vi "Compare Parameters.vi"(9 "refresh listbox":T4[](array[typedef]), 10 "new parameter":T1={"name"="", "unit"="", "Parameter"={"start index"=0, "size"=1, "encoding"=enum."BNR", "signed"=FALSE, "scale multiplier"=1.0, "scale offset"=0.0, "default value"=0.0}}, 11 "old parameter":T1={"name"="", "unit"="", "Parameter"={"start index"=0, "size"=1, "encoding"=enum."BNR", "signed"=FALSE, "scale multiplier"=1.0, "scale offset"=0.0, "default value"=0.0}}) -> (1 "refresh listbox out":T4[](array[typedef]), 2 "any changes?":bool)   [LabVIEW 2024, in "AIM ARINC 429 System Explorer.lvlib" / "Implementation.lvlib"]
uses:
  Implementation.lvlib
  Types/Refresh Listbox.ctl
  Types/Refresh Symbols.ctl
  Shared/VS Channel Definition for Parameter.ctl
  Shared/Parameter Definition.ctl
  <vilib>/NI/NI VeriStand Encoding and Decoding/Encoding.ctl
  Refresh Constants.vi
  <vilib>/NI/NI VeriStand Encoding and Decoding/Encoding and Decoding.lvlib
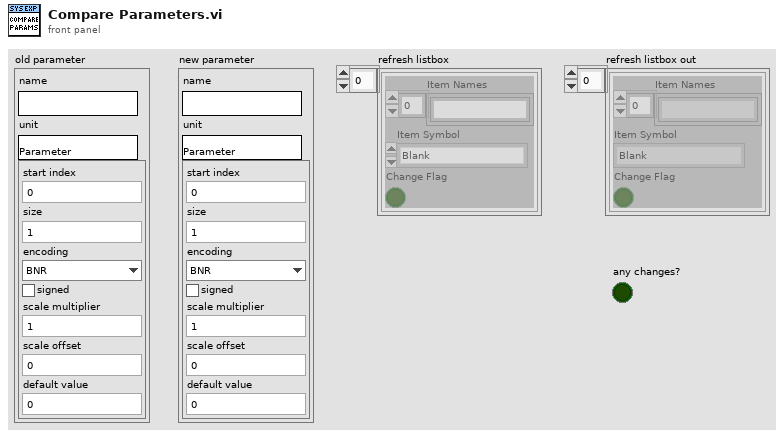
[diagram p1: front panel]
types:
  T1 = typedef "VS Channel Definition for Parameter.ctl" = cluster{"name":string, "unit":string, "Parameter":T2}
  T2 = typedef "Parameter Definition.ctl" = cluster{"start index":i32, "size":i32, "encoding":T3, "signed":bool, "scale multiplier":dbl, "scale offset":dbl, "default value":dbl}
  T3 = typedef "Encoding and Decoding.lvlib/Encoding.ctl" = enum16{"BNR", "BCD", "Discrete"}
  T4 = typedef "AIM ARINC 429 System Explorer.lvlib/Implementation.lvlib/Refresh Listbox.ctl" = cluster{"Item Names":string[], "Item Symbol":T5, "Change Flag":bool}
  T5 = typedef "AIM ARINC 429 System Explorer.lvlib/Implementation.lvlib/Refresh Symbols.ctl" = enum16{"Blank", "Port", "Incoming", "Outgoing", "Label", "Word", "Parameter", "ARINC-429", "Config Files", "Channel Spec", "Item"}
  T6 = cluster{"name":bool, "unit":bool, "Parameter":cluster{"start index":bool, "size":bool, "encoding":bool, "signed":bool, "scale multiplier":bool, "scale offset":bool, "default value":bool}}
  T7 = typedef "AIM ARINC 429 System Explorer.lvlib/Implementation.lvlib/Parameter Strings.ctl" = cluster{"name":string, "default value":string, "unit":string, "start index":string, "size":string, "encoding":string, "signed":string, "scale multiplier":string, "scale offset":string}
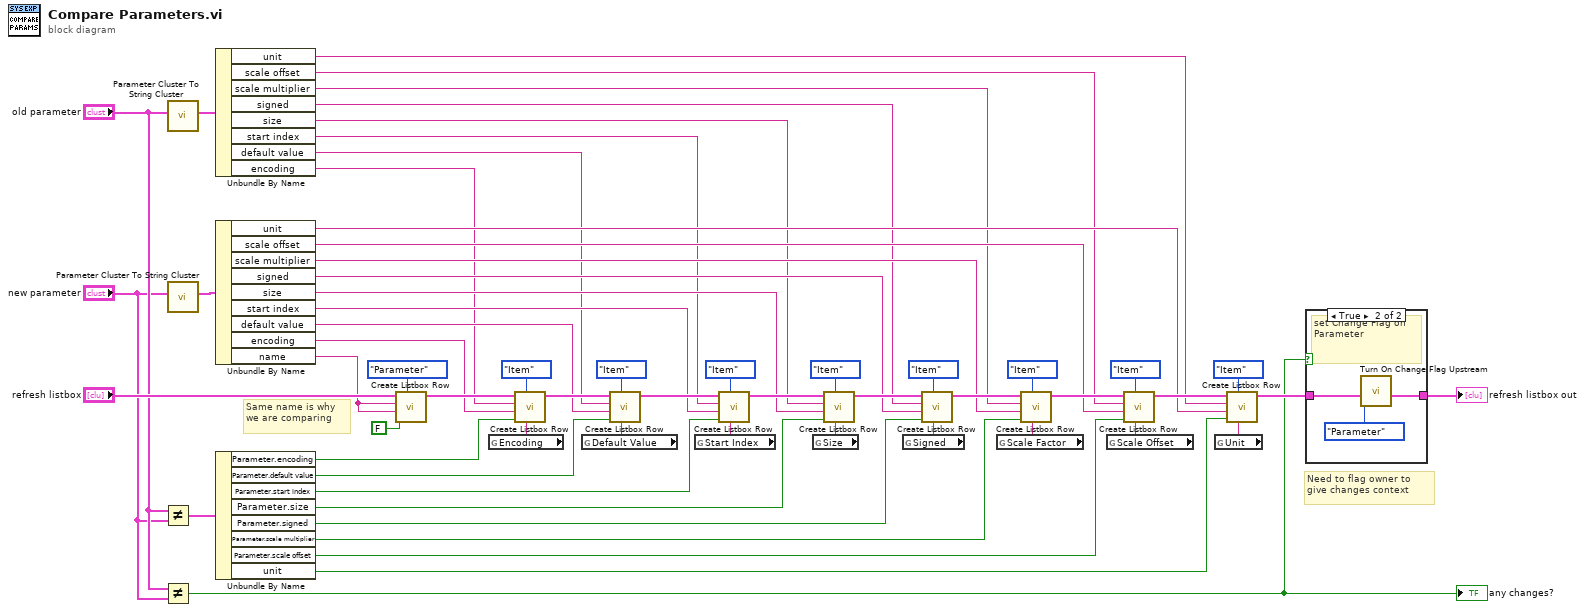
[diagram p0: block diagram]
diagram:
  # "Need to flag owner to give changes context"
  # "Same name is why we are comparing"
  n1 = Not Equal?(x="old parameter", y="new parameter") -> (x != y?=w14:T6)
  n2 = Not Equal?(x="old parameter", y="new parameter") -> (x != y?=w1:bool)
  "any changes?" <- w1
  n3 = call "Parameter Cluster To String Cluster.vi"("parameter"="old parameter") -> ("parameter strings"=w31:T7)  [unwired: 10 in]
  n4 = call "Parameter Cluster To String Cluster.vi"("parameter"="new parameter") -> ("parameter strings"=w41:T7)  [unwired: 10 in]
  n5 = Unbundle By Name(w31) -> ("unit"=w23:string, "scale offset"=w24:string, "scale multiplier"=w25:string, "signed"=w26:string, "size"=w27:string, "start index"=w28:string, "default value"=w29:string, "encoding"=w30:string)
  n6 = Unbundle By Name(w41) -> ("unit"=w32:string, "scale offset"=w33:string, "scale multiplier"=w34:string, "signed"=w35:string, "size"=w36:string, "start index"=w37:string, "default value"=w38:string, "encoding"=w39:string, "name"=w40:string)
  n7 = Unbundle By Name(w14) -> ("Parameter.encoding"=w13:bool, "Parameter.default value"=w12:bool, "Parameter.start index"=w11:bool, "Parameter.size"=w10:bool, "Parameter.signed"=w9:bool, "Parameter.scale multiplier"=w8:bool, "Parameter.scale offset"=w7:bool, "unit"=w6:bool)
  n8 = call "Create Listbox Row.vi"("refresh symbol (Blank)"=Refresh_Symbols."Parameter" ("Refresh Symbol (Blank)"), "change? (T)"=FALSE, "new item"=w40, "old item"=w40, "refresh listbox"="refresh listbox") -> ("refresh listbox out"=w57:T4[])  [unwired: 6 in]
  n9 = global read "Refresh Constants.vi" "Encoding"() -> (w22:string)
  n10 = call "Create Listbox Row.vi"("override name"=w22, "refresh symbol (Blank)"=Refresh_Symbols."Item" ("Refresh Symbol (Blank)"), "change? (T)"=w13, "new item"=w39, "old item"=w30, "refresh listbox"=w57) -> ("refresh listbox out"=w55:T4[])  [unwired: 5 in]
  n11 = global read "Refresh Constants.vi" "Default Value"() -> (w15:string)
  n12 = call "Create Listbox Row.vi"("override name"=w15, "refresh symbol (Blank)"=Refresh_Symbols."Item" ("Refresh Symbol (Blank)"), "change? (T)"=w12, "new item"=w38, "old item"=w29, "refresh listbox"=w55) -> ("refresh listbox out"=w53:T4[])  [unwired: 5 in]
  n13 = global read "Refresh Constants.vi" "Start Index"() -> (w16:string)
  n14 = call "Create Listbox Row.vi"("override name"=w16, "refresh symbol (Blank)"=Refresh_Symbols."Item" ("Refresh Symbol (Blank)"), "change? (T)"=w11, "new item"=w37, "old item"=w28, "refresh listbox"=w53) -> ("refresh listbox out"=w51:T4[])  [unwired: 5 in]
  n15 = global read "Refresh Constants.vi" "Size"() -> (w17:string)
  n16 = call "Create Listbox Row.vi"("override name"=w17, "refresh symbol (Blank)"=Refresh_Symbols."Item" ("Refresh Symbol (Blank)"), "change? (T)"=w10, "new item"=w36, "old item"=w27, "refresh listbox"=w51) -> ("refresh listbox out"=w49:T4[])  [unwired: 5 in]
  n17 = global read "Refresh Constants.vi" "Signed"() -> (w18:string)
  n18 = call "Create Listbox Row.vi"("override name"=w18, "refresh symbol (Blank)"=Refresh_Symbols."Item" ("Refresh Symbol (Blank)"), "change? (T)"=w9, "new item"=w35, "old item"=w26, "refresh listbox"=w49) -> ("refresh listbox out"=w47:T4[])  [unwired: 5 in]
  n19 = global read "Refresh Constants.vi" "Scale Factor"() -> (w19:string)
  n20 = call "Create Listbox Row.vi"("override name"=w19, "refresh symbol (Blank)"=Refresh_Symbols."Item" ("Refresh Symbol (Blank)"), "change? (T)"=w8, "new item"=w34, "old item"=w25, "refresh listbox"=w47) -> ("refresh listbox out"=w45:T4[])  [unwired: 5 in]
  n21 = global read "Refresh Constants.vi" "Scale Offset"() -> (w20:string)
  n22 = call "Create Listbox Row.vi"("override name"=w20, "refresh symbol (Blank)"=Refresh_Symbols."Item" ("Refresh Symbol (Blank)"), "change? (T)"=w7, "new item"=w33, "old item"=w24, "refresh listbox"=w45) -> ("refresh listbox out"=w43:T4[])  [unwired: 5 in]
  n23 = global read "Refresh Constants.vi" "Unit"() -> (w21:string)
  n24 = call "Create Listbox Row.vi"("override name"=w21, "refresh symbol (Blank)"=Refresh_Symbols."Item" ("Refresh Symbol (Blank)"), "change? (T)"=w6, "new item"=w32, "old item"=w23, "refresh listbox"=w43) -> ("refresh listbox out"=w5:T4[])  [unwired: 5 in]
  n25 = case shown="True" w1 {
    tunnel: w5 -> [w61 w64]
    tunnel: [w61 w62] -> w4
    frame False {
    }
    frame True {
      # "set Change Flag on Parameter"
      n26 = call "Turn On Change Flag Upstream.vi"("symbol to change"=Refresh_Symbols."Parameter", "refresh listbox"=w64) -> ("refresh listbox out"=w62:T4[])  [unwired: 9 in]
    }
  }
  "refresh listbox out" <- w4
